vi "Write sequencias.vi"(8 "error in (no error)":errorcluster, 10 "sequencias":u32, 11 "Channel in":refnum<class "Channel.lvclass">) -> (0 "error out":errorcluster, 3 "Channel out":refnum<class "Channel.lvclass">)   [LabVIEW 2018, in "Channel.lvclass"]
uses:
  Channel.lvclass
  Channel.lvclass/Channel.ctl
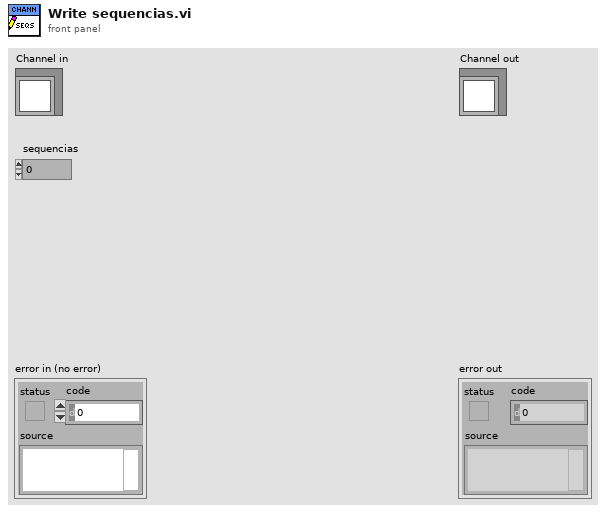
[diagram p1: front panel]
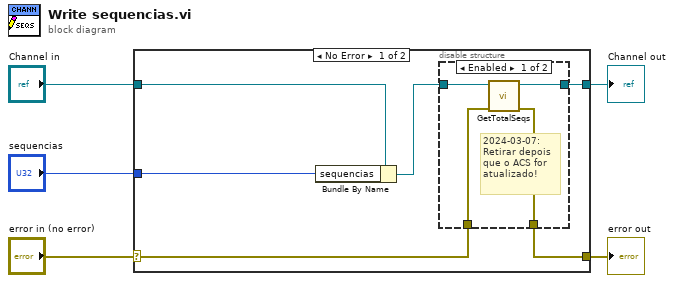
[diagram p0: block diagram]
diagram:
  n1 = case shown="No Error" "error in (no error)" {
    selector: "error in (no error)" -> [w8 w18]
    tunnel: [w6 w18] -> w4
    tunnel: [w7 w19] -> w2
    tunnel: "Channel in" -> [w11 w19]
    tunnel: "sequencias" -> [w10 _]
    frame No Error {
      n2 = Bundle By Name(cluster=w11, "sequencias"=w10) -> (w9:refnum<class "Channel.lvclass">)
      n3 = disable-structure shown="Enabled" {
        disable-tunnel: w9 -> [w15 w17]
        disable-tunnel: w8 -> [w14 w16]
        disable-tunnel: [w13 w17] -> w7
        disable-tunnel: [w12 w16] -> w6
        frame Enabled {
          # "2024-03-07:\nRetirar depois\nque o ACS for \natualizado!"
          n4 = call-dynamic "GetTotalSeqs.vi"("error in (no error)"=w14, "Channel in"=w15) -> ("error out"=w12:errorcluster, "Channel out"=w13:refnum<class "Channel.lvclass">)  [unwired: 8 in]
        }
        frame Disabled {
        }
      }
    }
    frame Error {
    }
  }
  "error out" <- w4
  "Channel out" <- w2
